vi "getNodeValue.vi"(8 "error in (no error)":errorcluster, 11 "NativeXML in":refnum<class "NativeXML.lvclass">) -> (0 "error out":errorcluster, 2 "Value":string, 3 "NativeXML out":refnum<class "NativeXML.lvclass">)   [LabVIEW 2009, in "Tools.lvlib" / "xml.lvlib" / "NativeXML.lvclass"]
uses:
  NativeXML.lvclass
  NativeXML.lvclass/NativeXML.ctl
  <vilib>/xml/NI_XML.lvlib
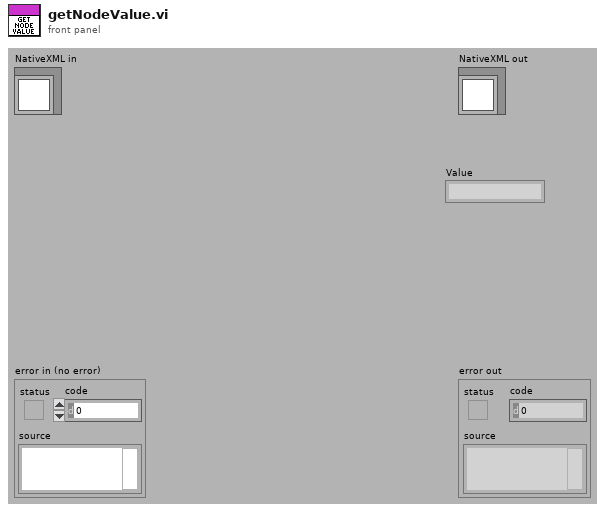
[diagram p1: front panel]
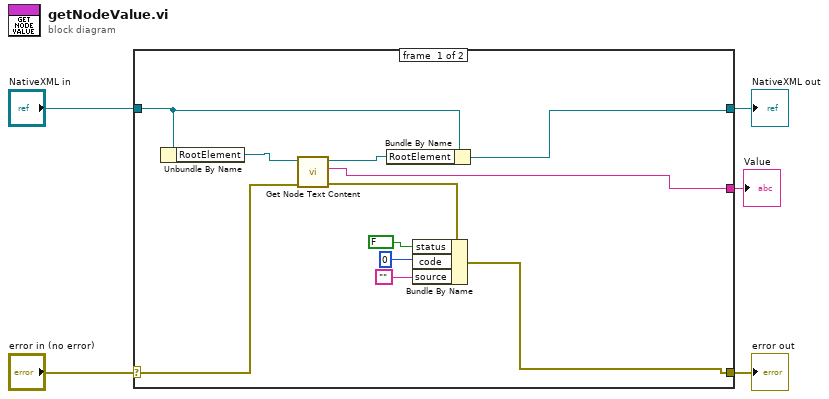
[diagram p0: block diagram]
diagram:
  n1 = case shown="No Error" "error in (no error)" {
    selector: "error in (no error)" -> [w12 w18]
    tunnel: [w6 w18] -> w4
    tunnel: [w15 w17] -> w2
    tunnel: "NativeXML in" -> [w16 w17]
    tunnel: [w11 _] -> w1
    frame #0 {
      n2 = Unbundle By Name(w16) -> ("RootElement"=w13:refnum<k20>)
      n3 = call <vilib>:"Get Node Text Content.vi"("error in (no error)"=w12, "node in"=w13) -> ("error out"=w10:errorcluster, "node text"=w11:string, "node out"=w14:refnum<k20>)  [unwired: 7 in]
      n4 = Bundle By Name(cluster=w16, "RootElement"=w14) -> (w15:refnum<class "NativeXML.lvclass">)
      n5 = Bundle By Name(cluster=w10, "status"=FALSE, "code"=0, "source"="") -> (w6:errorcluster)
    }
    frame #1 {
    }
  }
  "error out" <- w4
  "NativeXML out" <- w2
  "Value" <- w1
